vi "Trigger Detection for N Channel (obs).vi"(0 "signal in":waveform(dbl)[](array[waveform]), 1 "reset":bool, 5 "level":dbl[](array[numeric]) format="%0.2f", 7 "hysteresis":dbl[](array[numeric]) format="%0.2f", 9 "location mode":u16(ring) items=["Index", "Time"], 11 "error in (no error)":errorcluster, 12 "trigger slope":u16[](array[ring]) items=["Falling Edge", "Rising Edge"]) -> (4 "trigger locations":dbl[](array[numeric]) format="%0.2f", 8 "trigger detected?":bool[](array[boolean]), 15 "error out":errorcluster)   [LabVIEW 2020, in "NI_MAPro.lvlib"]
doc: "Finds the first level-crossing location in a waveform. You can retrieve the trigger location as an index or as a time. The trigger conditions are specified in terms of threshold <B>level</B>, <B>slope</B>, and <B>hysteresis</B>. The data type you wire to the <B>signal in</B> input determines the polymorphic instance to use."
uses:
  NI_MAPro.lvlib
  NI_MABase.lvlib
  <resource>/lvanlys.dll
panel:
  in  "max number trigger pts":i32=1
  out "final":dbl[](array[numeric]) format="%0.2f"
  out "number of triggers detected":i32[](array[numeric])
  out "triggerDetectedbyte":i32[](array[numeric])
  # "This VI is obsolete !!!\n\nNOTE: This obsolete VI uses the ending value in last data block as the instruction for the initial status of current data block. The new Trigger Detection VI uses the ending status instead."
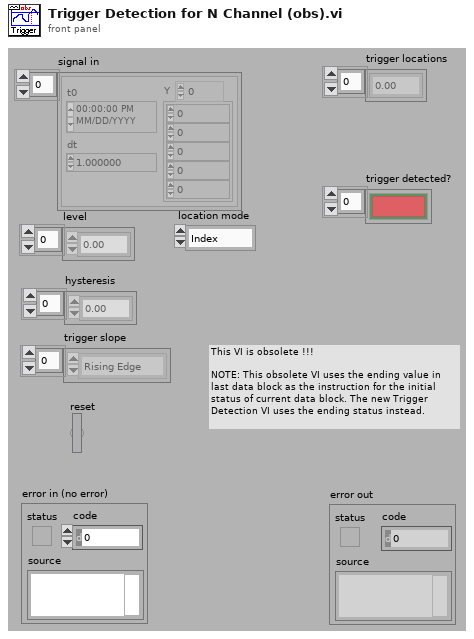
[diagram p1: front panel]
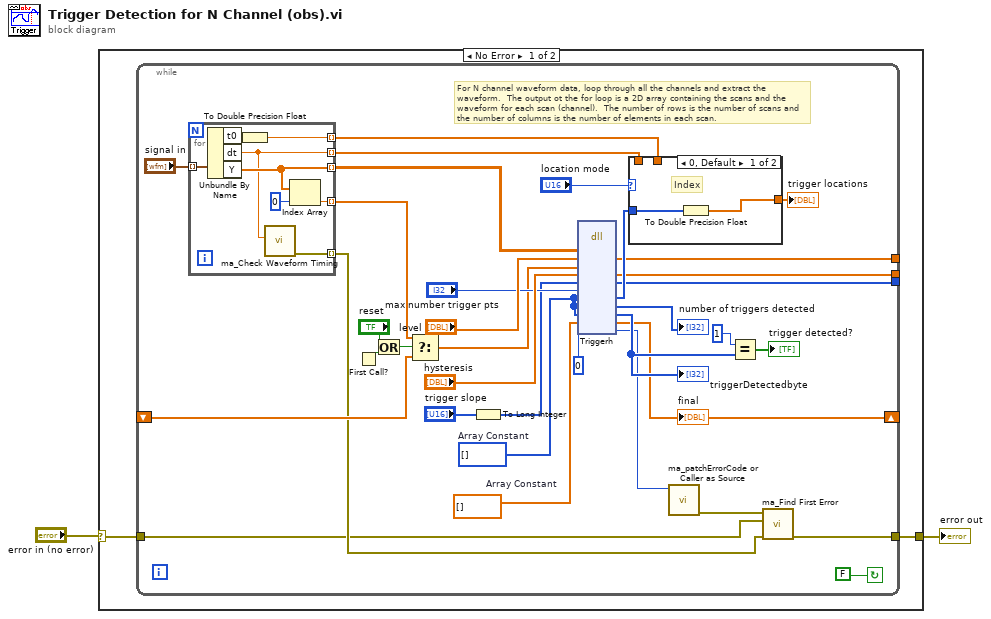
[diagram p0: block diagram]
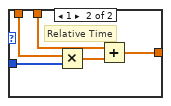
[diagram p2: hidden frame]
diagram:
  n1 = case shown="No Error" "error in (no error)" {
    selector: "error in (no error)" -> [w4 w55]
    tunnel: [w3 w55] -> w2
    frame No Error {
      n2 = while {
        tunnel: w4 -> [w11]
        tunnel: [w10] -> w3
        shift-right: [w13] -> _
        shift-left: _ -> [w24]
        tunnel: [w7] -> _
        tunnel: [w6] -> _
        tunnel: [w5] -> _
        stop <- FALSE continue-if-true
        w33 = dbl[] []  # Array Constant
        w16 = i32[] []  # Array Constant
        # "For N channel waveform data, loop through all the channels and extract the waveform.  The output ot the for loop is a 2D array containing the scans and the waveform for each scan (channel).  The number of rows is the number of scans and the number of columns is the number of elements in each scan."
        n3 = for {
          tunnel: "signal in" -> [w54] mode=indexing
          tunnel: [w53] -> w38 mode=indexing
          tunnel: [w51] -> w25 mode=indexing
          tunnel: [w48] -> w18 mode=indexing
          tunnel: [w50] -> w17 mode=indexing
          tunnel: [w47] -> w12 mode=indexing
          n4 = Unbundle By Name(w54) -> ("t0"=w49:timestamp, "dt"=w48:dbl, "Y"=w53:dbl[])
          n5 = To Double Precision Float(number=w49) -> (double precision float=w50:dbl)
          n6 = call "ma_Check Waveform Timing.vi"("dt"=w48) -> ("error out"=w47:errorcluster)  [unwired: 2 in, 8 out]
          n7 = Index Array(array=w53, index=0 ("Index")) -> (element=w51:dbl)
        }
        n8 = First Call?() -> (First Call?: T/F=w15:bool)
        n9 = Or(x="reset", y=w15) -> (x .or. y?=w26:bool)
        n10 = Select(t=w25, s=w26, f=w24) -> (s? t:f=w23:dbl[])
        n11 = To Long Integer(number="trigger slope") -> (32bit integer=w22:i32[])
        n12 = dll-call lib="C:/Program Files (x86)/National Instruments/LabVIEW 2020/resource/lvanlys.*" fn="Triggerh"("x"=w38, "level"="level", "initial"=w23, "hysterisis"="hysteresis", "slope"=w22, "ntptsH"="max number trigger pts", "triggerIndex"=w16, "number_of_triggers_detected"=w16, "triggerDetectedbyte"=w16, "final"=w33, "error"=0) -> ("level"=w7:dbl[], "hysterisis"=w6:dbl[], "slope"=w5:i32[], "triggerIndex"=w20:i32[], "number_of_triggers_detected"=→"number of triggers detected":i32[], "triggerDetectedbyte"=w30:i32[], "final"=w13:dbl[], "error"=w9:i32)  [unwired: 6 in, 3 out]
        "triggerDetectedbyte" <- w30
        "final" <- w13
        n13 = case shown="0, Default" "location mode" {
          tunnel: w20 -> [w41 w46]
          tunnel: [w40 w43] -> w19
          tunnel: w18 -> [_ w45]
          tunnel: w17 -> [_ w42]
          frame 0, Default {
            # "Index"
            n14 = To Double Precision Float(number=w41) -> (double precision float=w40:dbl[])
          }
          frame 1 {
            # "Relative Time"
            n15 = Multiply(x=w45, y=w46) -> (x*y=w44:dbl[])
            n16 = Add(x=w42, y=w44) -> (x+y=w43:dbl[])
          }
        }
        "trigger locations" <- w19
        n17 = call "ma_patchErrorCode or Caller as Source.vi"("error code"=w9) -> ("error out"=w8:errorcluster)  [unwired: 3 in, 7 out]
        n18 = Equal?(x=u8 1 ("Element Data"), y=w30) -> (x = y?=→"trigger detected?":bool[])
        n19 = call "ma_Find First Error.vi"("error array in"=w12, "error in 2 (no error)"=w11, "error in 1 (no error)"=w8) -> ("error out"=w10:errorcluster)  [unwired: 1 in, 3 out]
      }
    }
    frame Error {
    }
  }
  "error out" <- w2
